vi "escapi_capture_image.vi"(8 "error in (no error)":errorcluster, 10 "identifier":string, 11 "Image in":T1) -> (0 "error out":errorcluster, 3 "Image out":T1)   [LabVIEW 2022 SP3, in "Vision.lvlib"]
uses:
  Vision.lvlib
  <vilib>/vision/Image Controls.llb/IMAQ Image.ctl
  bin/Vision.dll
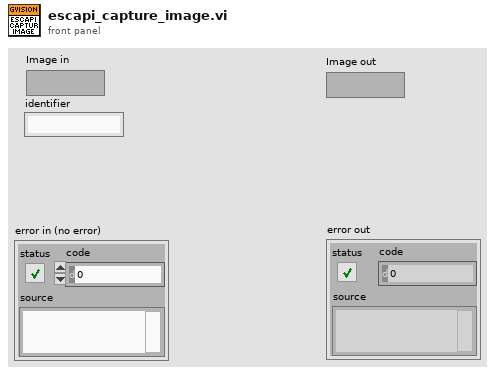
[diagram p1: front panel]
types:
  T1 = typedef "IMAQ Image.ctl" = refnum<image>
  T2 = enum32{"Map Pixel Pointer", "Unmap Pixel Pointer", "Get Pixels Infos"}
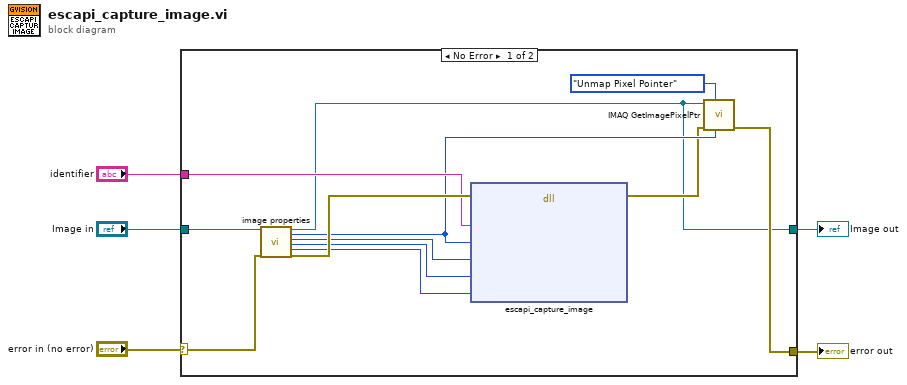
[diagram p0: block diagram]
diagram:
  n1 = case shown="No Error" "error in (no error)" {
    selector: "error in (no error)" -> [w16 w19]
    tunnel: [w8 w19] -> w4
    tunnel: "Image in" -> [w17 w18]
    tunnel: "identifier" -> [w14 _]
    tunnel: [w6 w18] -> w1
    frame No Error {
      n2 = call "image properties.vi"("Image in"=w17, "error in (no error)"=w16) -> ("Image out"=w6:T1, "Pixel Pointer out"=w10:u64, "Line Width"=w13:i32, "X Resolution"=w12:i32, "Y Resolution"=w11:i32, "error out"=w15:errorcluster)  [unwired: 10 in, 2 out]
      n3 = dll-call lib="C:/Users/Caleb/Desktop/nebraska-silicon-lab/pixel-gantry-extra/LV/bin/Vision.dll" fn="escapi_capture_image"(error in=w15, "camera_name"=w14, "dstPtr"=w10, "dstLineWidth"=w13, "dstWidth"=w12, "dstHeight"=w11) -> (error out=w9:errorcluster)  [unwired: 8 in, 1 out]
      n4 = call "IMAQ GetImagePixelPtr"("Pixel Pointer in"=w10, "Function"=T2."Unmap Pixel Pointer", "error in (no error)"=w9, "Image"=w6) -> ("error out"=w8:errorcluster)  [unwired: 2 in, 5 out]
    }
    frame Error {
    }
  }
  "error out" <- w4
  "Image out" <- w1
